vi "SphericalStripLIM.vi"() -> ()   [LabVIEW 2022 SP3]
uses:
  <vilib>/Platform/NI_3dgraph.lvlib
  <vilib>/measure/NI_MABase.lvlib
panel:
  in  "Ring":u16(ring) items=["Strip", "sphere section"]
  in  "number of rim points":i32=200
  in  "3D Surface":refnum<k7>(container)
  in  "Points":i32=10
  in  "Plane":u16(ring)=2 items=["X-Y", "Y-Z", "Z-X"]
  in  "P (cm)":cluster{"x":dbl, "y":dbl, "z":dbl}={"x"=4.0, "y"=0.0, "z"=4.0} {"x" format="%.2f"; "z" format="%.2f"; "y" format="%.2f"}
  in  "strip (cm)":cluster{"radius":dbl, "h":dbl, "w":dbl}={"radius"=10.0, "h"=5.0, "w"=4.0} {"radius" format="%.2f"; "w" format="%.2f"; "h" format="%.2f"}
  # "Use line integral method to solve for pressure wave form."
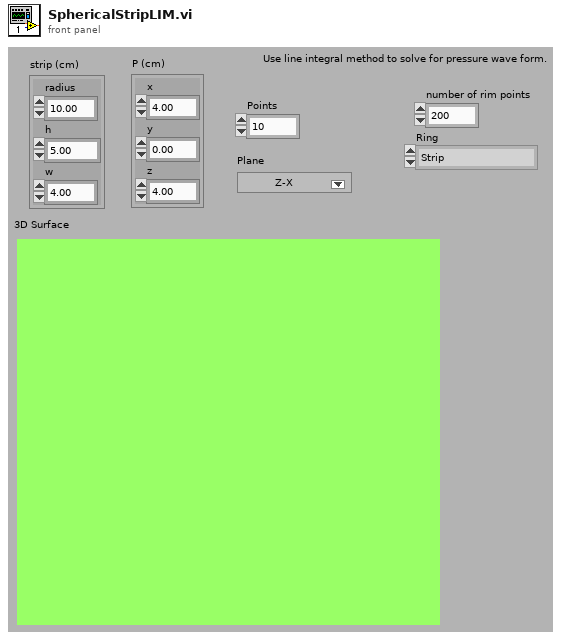
[diagram p1: front panel]
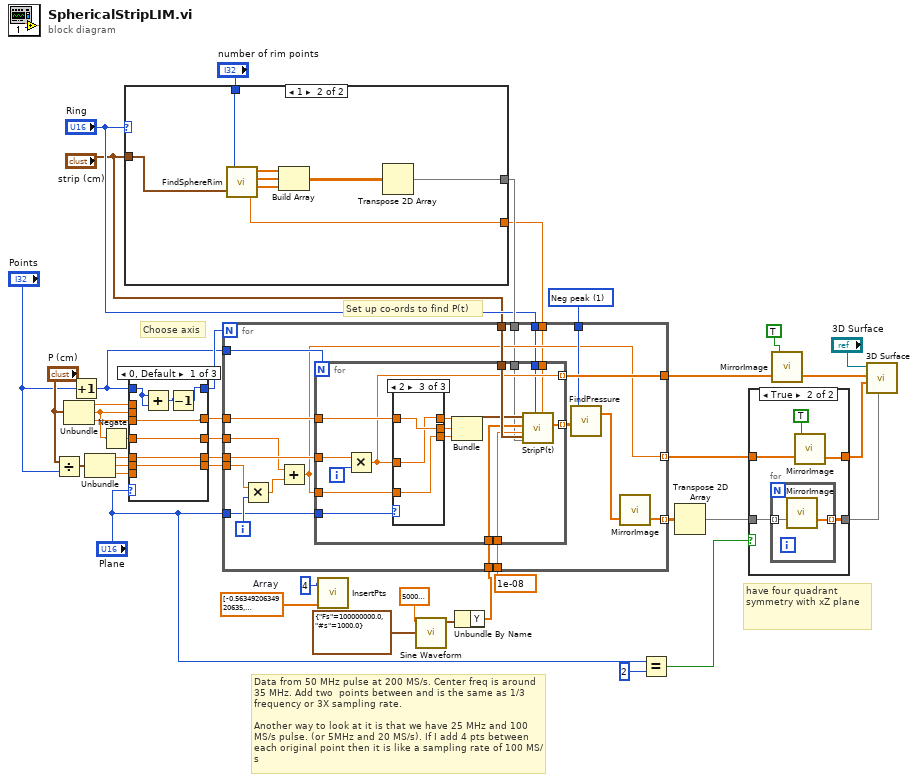
[diagram p0: block diagram]
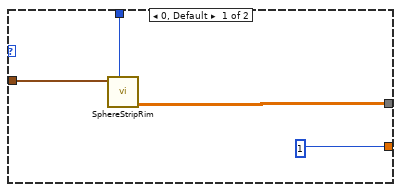
[diagram p2: hidden frame]
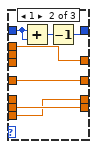
[diagram p4: hidden frame]
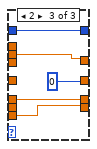
[diagram p5: hidden frame]
diagram:
  w23 = u16 1 items=["Pos Peak", "Neg peak", "Steady State"] ("Pressure Calc")
  w6 = dbl[] [-0.5634920634920635, -0.6825396825396826, -0.8015873015873016, -0.9920634920634921, -1.1507936507936507, -1.3888888888888888, -1.992063492063492, -4.2063492063492065, -5.888888888888889, 13.023809523809524, 61.32539682539682, 92.83333333333333, 75.10317460317461, 18.126984126984127, -54.93650793650794, -109.60317460317461, -104.22222222222223, 18.134920634920636, 83.33333333333333, 27.27777777777778, -42.19047619047619, -45.63492063492063, 10.15079365079365, 49.05555555555556, 28.19047619047619, -5.658730158730159, -15.261904761904763, -4.4603174603174605, 7.984126984126984, 10.682539682539682, 5.809523809523809, -0.03968253968253968, -2.515873015873016, -1.4841269841269842, 1.0396825396825398, 2.0555555555555554, 0.9523809523809523, -0.6031746031746031, -1.007936507936508, -0.3968253968253968, 0.14285714285714285]  # Array
  # "have four quadrant symmetry with xZ plane"
  # "Set up co-ords to find P(t)"
  # "Choose axis"
  # "Data from 50 MHz pulse at 200 MS/s. Center freq is around 35 MHz. Add two  points between and is the same as 1/3 frequency or 3X sampling rate.\n\nAnother way to look at it is that we have 25 MHz and 100 MS/s pulse. (or 5MHz and 20 MS/s). If I add 4 pts between each original point then it is like a sampling rate of 100 MS/s"
  n1 = Divide(x="P (cm)", y="Points") -> (x/y=w38:cluster{"x":dbl, "y":dbl, "z":dbl})
  n2 = Unbundle("P (cm)") -> ("x"=w40:dbl, "y"=w28:dbl, "z"=w39:dbl)
  n3 = Increment(x="Points") -> (x+1=w8:i32)
  n4 = Unbundle(w38) -> ("x"=w37:dbl, "y"=w35:dbl, "z"=w32:dbl)
  n5 = Negate(x=w28) -> (-x=w20:dbl)
  n6 = case shown="1" "Ring" {
    tunnel: "number of rim points" -> [w45 w51]
    tunnel: "strip (cm)" -> [w44 w52]
    tunnel: [w43 w50] -> w12
    tunnel: [1 w49] -> w7
    frame 0, Default {
      n7 = call "SphereStripRim.vi"("number of points"=w45, "Ducer"=w44) -> ("rim points"=w43:dbl[][])  [unwired: 8 in]
    }
    frame 1 {
      n8 = call "FindSphereRim.vi"("number of rim points"=w51, "strip (cm)"=w52) -> ("x"=w46:dbl[], "y"=w47:dbl[], "z"=w48:dbl[], "d"=w49:dbl)
      n9 = Build Array(w46, w47, w48) -> (w53:dbl[][])
      n10 = Transpose 2D Array(2D array=w53) -> (transposed array=w50:dbl[][])
    }
  }
  n11 = case shown="0, Default" "Plane" {
    tunnel: w40 -> [_ w67 _]
    tunnel: w28 -> [_ _ w72]
    tunnel: w39 -> [w58 _ _]
    tunnel: [w60 w63 w71] -> w36
    tunnel: w37 -> [w60 _ w71]
    tunnel: [w59 w64 w70] -> w34
    tunnel: w35 -> [w59 w64 _]
    tunnel: [w58 w67 w72] -> w33
    tunnel: w32 -> [_ w63 w70]
    tunnel: w8 -> [w57 w66 w69]
    tunnel: [w54 w61 w69] -> w29
    tunnel: [w56 w62 0] -> w19
    tunnel: w20 -> [w56 w62 _]
    frame 0, Default {
      n12 = Add(x=w57, y=w57) -> (x+y=w55:i32)
      n13 = Decrement(x=w55) -> (x-1=w54:i32)
    }
    frame 1 {
      n14 = Add(x=w66, y=w66) -> (x+y=w65:i32)
      n15 = Decrement(x=w65) -> (x-1=w61:i32)
    }
    frame 2 {
    }
  }
  n16 = call "InsertPts.vi"("Array in"=w6, "pts to insert"=4) -> ()  [unwired: 1 out]
  n17 = call <vilib>:"Sine Waveform.vi"("sampling info"=cluster{"Fs":dbl, "#s":dbl} {"Fs"=100000000.0, "#s"=1000.0}, "frequency"=5000000.0) -> ("signal out"=w4:waveform(dbl))  [unwired: 8 in, 1 out]
  n18 = Unbundle By Name(w4) -> ("Y"=w1:dbl[])
  n19 = for {
    N: w29 -> [_]
    tunnel: w36 -> [w91]
    tunnel: w34 -> [w90]
    tunnel: w33 -> [w89]
    tunnel: "strip (cm)" -> [w88]
    tunnel: w1 -> [w87]
    tunnel: 1e-08 ("waveform sampling rate 1/2)") -> [w86]
    tunnel: "Plane" -> [w84]
    tunnel: [w77] -> w22 mode=indexing
    tunnel: w8 -> [w83]
    tunnel: w19 -> [w80]
    tunnel: [w82] -> w18
    tunnel: w23 -> [w81]
    tunnel: [w78] -> w17 mode=indexing
    tunnel: w12 -> [w75]
    tunnel: "Ring" -> [w74]
    tunnel: w7 -> [w73]
    i -> [w92]
    n20 = Multiply(x=w90, y=w92) -> (x*y=w79:dbl)
    n21 = Add(x=w80, y=w79) -> (x+y=w78:dbl)
    n22 = for {
      N: w83 -> [_]
      tunnel: w91 -> [w108]
      tunnel: w89 -> [w107]
      tunnel: w78 -> [w103]
      tunnel: w88 -> [w102]
      tunnel: w87 -> [w101]
      tunnel: w86 -> [w100]
      tunnel: [w99] -> w85 mode=indexing
      tunnel: w84 -> [w98]
      tunnel: [w97] -> w82 mode=indexing
      tunnel: w75 -> [w95]
      tunnel: w74 -> [w94]
      tunnel: w73 -> [w93]
      i -> [w109]
      n23 = Multiply(x=w108, y=w109) -> (x*y=w97:dbl)
      n24 = case shown="2" w98 {
        tunnel: [w111 w115 w117] -> w106
        tunnel: w107 -> [w112 w115 w118]
        tunnel: [w112 w113 w116] -> w105
        tunnel: [w110 w114 w118] -> w104
        tunnel: w103 -> [w110 w114 w116]
        tunnel: w97 -> [w111 w113 w117]
        frame 0, Default {
        }
        frame 1 {
        }
        frame 2 {
        }
      }
      n25 = Bundle("y"=w106, "y"=w104, "y"=w105) -> (w96:cluster{"y":dbl, "y":dbl, "y":dbl})  [unwired: 1 in]
      n26 = call "StripP(t).vi"("d (depth of curvature)"=w93, "strip (cm)"=w102, "Ring"=w94, "edge points"=w95, "waveform sampling rate s"=w100, "drive signal"=w101, "P (cm)"=w96) -> ("Waveform Graph"=w99:dbl[])  [unwired: 3 in, 1 out]
    }
    n27 = call "FindPressure.vi"("Input"=w85, "Pressure Calc"=w81) -> ("Pressures"=w76:dbl[])  [unwired: 1 in]
    n28 = call "MirrorImage.vi"("input"=w76) -> ("output"=w77:dbl[])  [unwired: 2 in]
  }
  n29 = Equal?(x="Plane", y=2) -> (x = y?=w25:bool)
  n30 = Transpose 2D Array(2D array=w22) -> (transposed array=w16:dbl[][])
  n31 = case shown="True" w25 {
    tunnel: [w120 w125] -> w5
    tunnel: w16 -> [w120 w124]
    tunnel: w17 -> [w119 w121]
    tunnel: [w119 w122] -> w14
    frame False {
    }
    frame True {
      n32 = for {
        tunnel: w124 -> [w127] mode=indexing
        tunnel: [w126] -> w125 mode=indexing
        n33 = call "MirrorImage.vi"("input"=w127) -> ("output"=w126:dbl[])  [unwired: 2 in]
      }
      n34 = call "MirrorImage.vi"("input"=w121, "neg?"=TRUE) -> ("output"=w122:dbl[])  [unwired: 1 in]
    }
  }
  n35 = call "MirrorImage.vi"("input"=w18, "neg?"=TRUE) -> ("output"=w15:dbl[])  [unwired: 1 in]
  n36 = call <vilib>:"3D Surface.vi"("z matrix"=w5, "y vector"=w14, "x vector"=w15, "3D graph"="3D Surface") -> ()  [unwired: 6 in, 2 out]
